vi "Init.Python.vi"   [LabVIEW 2014]
uses:
  python27.dll
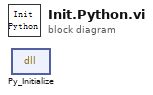
[diagram p0: block diagram]
diagram:
  n1 = dll-call lib="python27.dll" fn="Py_Initialize"() -> ()  [unwired: 4 in, 2 out]
